vi "zegar.vi"(1 "zadanie":enum16{"Start", "Pauza", "Pomiar"}(ring)=enum."Pomiar") -> (0 "x-y":dbl)   [LabVIEW 2018]
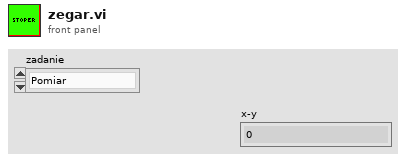
[diagram p1: front panel]
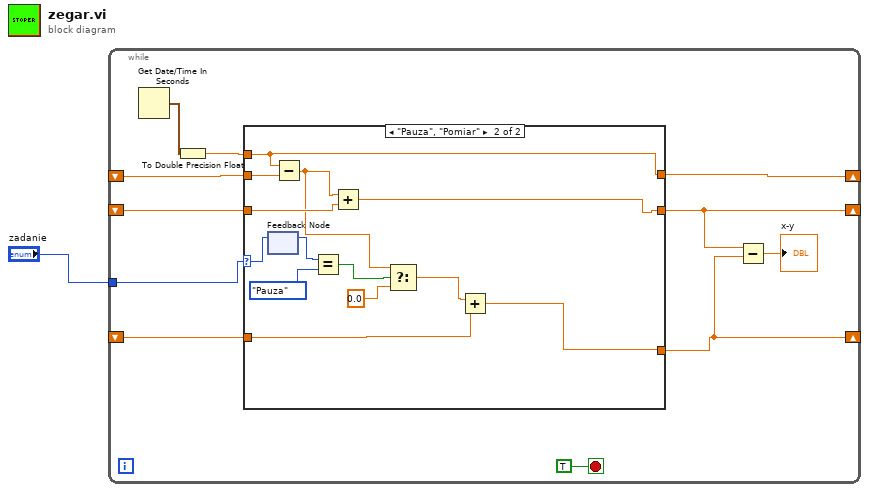
[diagram p0: block diagram]
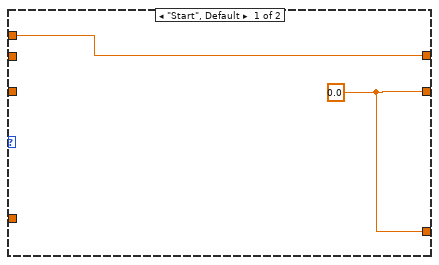
[diagram p2: hidden frame]
diagram:
  n1 = while {
    shift-right: [w5] -> _
    shift-left: _ -> [w11]
    shift-right: [w8] -> _
    shift-left: _ -> [w7]
    shift-right: [w4] -> _
    shift-left: _ -> [w6]
    tunnel: "zadanie" -> [w2]
    stop <- TRUE stop-if-true
    n2 = Get Date/Time In Seconds() -> (seconds since 1Jan1904=w10:timestamp)
    n3 = To Double Precision Float(number=w10) -> (double precision float=w9:dbl)
    n4 = case shown="\"Pauza\", \"Pomiar\"" w2 {
      selector: w2 -> [_ w16]
      tunnel: w11 -> [_ w26]
      tunnel: [w13 w25] -> w5
      tunnel: w9 -> [w14 w24]
      tunnel: [w14 w24] -> w8
      tunnel: w7 -> [_ w27]
      tunnel: w6 -> [_ w18]
      tunnel: [w13 w17] -> w4
      frame "Start", Default {
        w13 = 0.0
      }
      frame "Pauza", "Pomiar" {
        n5 = feedback-in #1(w16) -> ()
        n6 = feedback #1() -> (w15:enum16{"Start", "Pauza", "Pomiar"})  [unwired: 1 in]
        n7 = Subtract(x=w24, y=w27) -> (x-y=w20:dbl)
        n8 = Equal?(x=w15, y=enum16{"Start", "Pauza", "Pomiar"}."Pauza") -> (x = y?=w22:bool)
        n9 = Add(x=w20, y=w26) -> (x+y=w25:dbl)
        n10 = Select(t=w20, s=w22, f=0.0) -> (s? t:f=w19:dbl)
        n11 = Add(x=w19, y=w18) -> (x+y=w17:dbl)
      }
    }
    n12 = Subtract(x=w5, y=w4) -> (x-y=→"x-y":dbl)
  }
